vi "DP-Assign Speakers.vi"(0 "Primary":path, 1 "F1 Max Req":dbl, 2 "F2 Max  Req":dbl, 5 "Secondary":path, 9 "freq":dbl[](array[numeric]), 11 "error in (no error)":errorcluster) -> (4 "Flipped?":bool, 10 "Nominal Max SPL":dbl[](array[numeric]), 15 "error out":errorcluster)   [LabVIEW 2020]
uses:
  862417d9-73a4-4875-ab11-c892e595ea43.vi
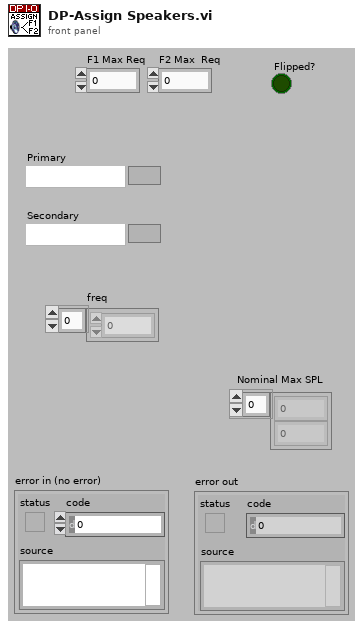
[diagram p1: front panel]
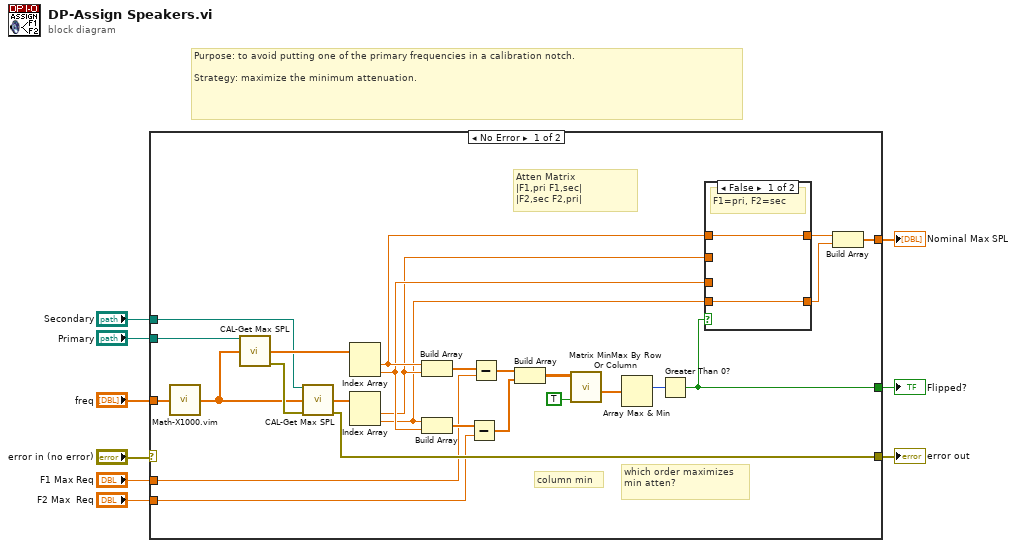
[diagram p0: block diagram]
diagram:
  # "Purpose: to avoid putting one of the primary frequencies in a calibration notch.\n\nStrategy: maximize the minimum attenuation."
  n1 = case shown="No Error" "error in (no error)" {
    selector: "error in (no error)" -> [_ w40]
    tunnel: [w30 w40] -> w8
    tunnel: [w24 _] -> w7
    tunnel: "F1 Max Req" -> [w23 _]
    tunnel: "F2 Max  Req" -> [w22 _]
    tunnel: [w15 _] -> w4
    tunnel: "Primary" -> [w14 _]
    tunnel: "Secondary" -> [w13 _]
    tunnel: "freq" -> [w12 _]
    frame No Error {
      # "which order maximizes min atten?"
      # "column min"
      # "Atten Matrix\n|F1,pri F1,sec|\n|F2,sec F2,pri|"
      n2 = call "Math-X1000.vim"("X"=w12) -> ("1000X"=w10:dbl[])
      n3 = call "CAL-Get Max SPL.vi"("Speaker name"=w14, "Frequency (Hz)"=w10) -> ("Max SPL"=w34:dbl[], "error out"=w35:errorcluster)  [unwired: 12 in]
      n4 = call "CAL-Get Max SPL.vi"("Speaker name"=w13, "Frequency (Hz)"=w10, "error in (no error)"=w35) -> ("Max SPL"=w33:dbl[], "error out"=w30:errorcluster)  [unwired: 11 in]
      n5 = Index Array(array=w34) -> (element #1=w21:dbl, element #2=w20:dbl)  [unwired: 2 in]
      n6 = Index Array(array=w33) -> (element #1=w19:dbl, element #2=w18:dbl)  [unwired: 2 in]
      n7 = Build Array(w21, w19) -> (w32:dbl[])
      n8 = Build Array(w18, w20) -> (w31:dbl[])
      n9 = Subtract(x=w31, y=w22) -> (x-y=w28:dbl[])
      n10 = Subtract(x=w32, y=w23) -> (x-y=w29:dbl[])
      n11 = Build Array(w29, w28) -> (w27:dbl[][])
      n12 = call "Matrix MinMax By Row Or Column.vi"("By column?"=TRUE, "2D Array"=w27) -> ("Min Vector"=w26:dbl[])  [unwired: 6 in, 3 out]
      n13 = Array Max & Min(array=w26) -> (max index (indices)=w25:i32)  [unwired: 3 out]
      n14 = Greater Than 0?(x=w25) -> (x > 0?=w24:bool)
      n15 = case shown="False" w24 {
        tunnel: w21 -> [w37 _]
        tunnel: w20 -> [_ w38]
        tunnel: w19 -> [_ w39]
        tunnel: [w37 w39] -> w16
        tunnel: w18 -> [w36 _]
        tunnel: [w36 w38] -> w17
        frame False {
          # "F1=pri, F2=sec"
        }
        frame True {
          # "F1=sec; F2=pri"
        }
      }
      n16 = Build Array(w16, w17) -> (w15:dbl[])
    }
    frame Error {
    }
  }
  "error out" <- w8
  "Flipped?" <- w7
  "Nominal Max SPL" <- w4
